vi "while loop sevo control.vi"() -> ()   [LabVIEW 2022 SP3]
uses:
  <vilib>/DAQmx/write.llb/DAQmx Write (Digital Bool 1Line 1Point).vi
  <vilib>/DAQmx/create/channels.llb/DAQmx Create Channel (DO-Digital Output).vi
  <vilib>/DAQmx/miscellaneous.llb/DAQmx Fill In Error Info.vi
panel:
  in  "Slide":dbl(slide) scale=1.0..2.0
  in  "stop":bool
  in  "lines 2":tag
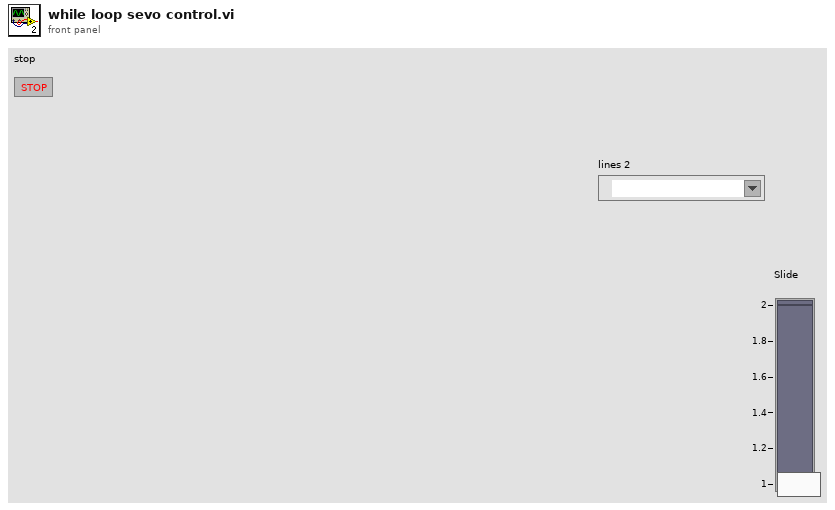
[diagram p1: front panel]
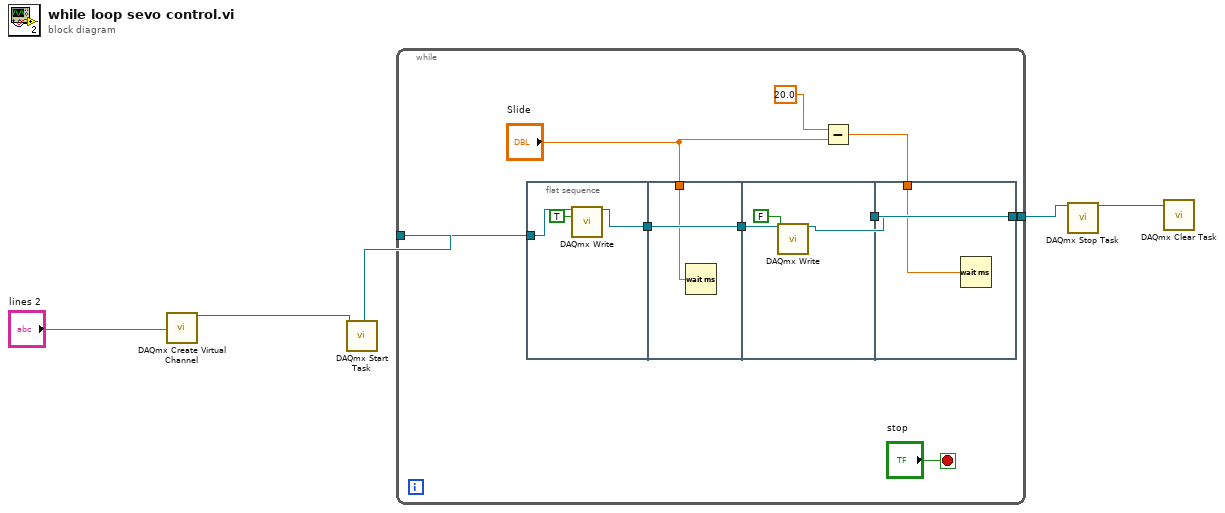
[diagram p0: block diagram]
diagram:
  n1 = call-poly <vilib>:"DAQmx Create Virtual Channel.vi"("lines"="lines 2") -> ("task out"=w4:refnum<k21>)  [unwired: 13 in, 1 out]
  n2 = call <vilib>:"DAQmx Start Task.vi"("task/channels in"=w4) -> ("task out"=w3:refnum<k21>)  [unwired: 13 in, 1 out]
  n3 = while {
    tunnel: w3 -> [w14]
    tunnel: [w11] -> w1
    stop <- "stop" stop-if-true
    n4 = flat-sequence {
      tunnel: w14 -> [w17]
      tunnel: [w16] -> w12
      tunnel: [w19] -> w13
      tunnel: w12 -> [w19]
      tunnel: "Slide" -> [w18]
      tunnel: w13 -> [w21]
      tunnel: [w22] -> w9
      tunnel: [w24] -> w11
      tunnel: w9 -> [w24]
      tunnel: w6 -> [w23]
      frame #0 {
        n5 = call-poly <vilib>:"DAQmx Write.vi"("task/channels in"=w17, "data"=TRUE) -> ("task out"=w16:refnum<k21>)  [unwired: 11 in, 2 out]
      }
      frame #1 {
        n6 = Wait (ms)(milliseconds to wait=w18) -> ()  [unwired: 1 out]
      }
      frame #2 {
        n7 = call-poly <vilib>:"DAQmx Write.vi"("task/channels in"=w21, "data"=FALSE) -> ("task out"=w22:refnum<k21>)  [unwired: 11 in, 2 out]
      }
      frame #3 {
        n8 = Wait (ms)(milliseconds to wait=w23) -> ()  [unwired: 1 out]
      }
    }
    n9 = Subtract(x=20.0, y="Slide") -> (x-y=w6:dbl)
  }
  n10 = call <vilib>:"DAQmx Stop Task.vi"("task/channels in"=w1) -> ("task out"=w2:refnum<k21>)  [unwired: 13 in, 1 out]
  n11 = call <vilib>:"DAQmx Clear Task.vi"("task in"=w2) -> ()  [unwired: 14 in, 1 out]
